vi "Write Default Value.vi"(8 "error in":errorcluster, 10 "default value":bool, 11 "digital channel in":refnum<class "Digital Channel.lvclass">) -> (0 "error out":errorcluster, 3 "digital channel out":refnum<class "Digital Channel.lvclass">)   [LabVIEW 2020, in "Scan Engine Scripting.lvlib" / "Digital Channel.lvclass"]
uses:
  Digital Channel.lvclass
  Digital Channel.lvclass/Digital Channel.ctl
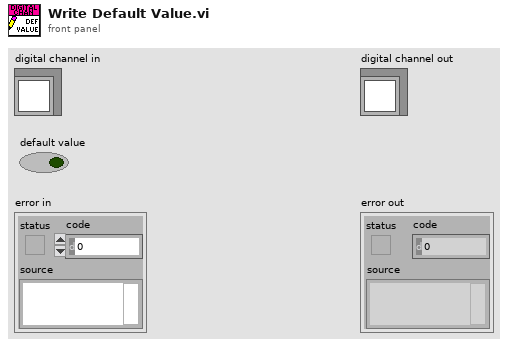
[diagram p1: front panel]
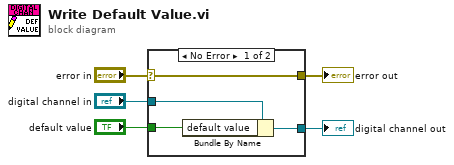
[diagram p0: block diagram]
diagram:
  n1 = case shown="No Error" "error in" {
    selector: "error in" -> [w9 w10]
    tunnel: [w9 w10] -> w4
    tunnel: [w7 w11] -> w2
    tunnel: "digital channel in" -> [w8 w11]
    tunnel: "default value" -> [w6 _]
    frame No Error {
      n2 = Bundle By Name(cluster=w8, "default value"=w6) -> (w7:refnum<class "Digital Channel.lvclass">)
    }
    frame Error {
    }
  }
  "error out" <- w4
  "digital channel out" <- w2
